vi "Get QControl Class Hierarchy.vi"(11 "ControlClassWizard in":refnum<class "QControl Creation Wizard.lvclass">) -> (0 "error out":errorcluster, 2 "QControl Class Hierarchy":string[][](array[string]), 3 "ControlClassWizard out":refnum<class "QControl Creation Wizard.lvclass">)   [LabVIEW 2015, in "QControl Creation Wizard.lvclass"]
doc: "<b> </b> <b> </b>\n©2016 Q Software Innovations, LLC (QSI)\nwritten by Quentin Alldredge\nproduced in LabVIEW 2015\n\nsupport@qsoftwareinnovations.com\nwww.qsoftwareinnovations.com\n\nAll rights reserved.\n\nRedistribution and use in source and binary forms, with or without modification, are permitted provided that the following conditions are met:\n\n * Redistributions of source code must retain the above copyright notice, this list of conditions and the following disclaimer.\n * Redistributions in binary form must reproduce the above copyright notice, this list of conditions and the following disclaimer in the documentation and/or other materials provided with the distribution.\n * Neither the name of Q Software Innovations, LLC. nor the names of its contributors may be used to endorse or promote products derived from this software without specific prior written permission.\n\nTHIS SOFTWARE IS PROVIDED BY THE COPYRIGHT HOLDERS AND CONTRIBUTORS \"AS IS\" AND ANY EXPRESS OR IMPLIED WARRANTIES, INCLUDING, BUT NOT LIMITED TO, THE IMPLIED WARRANTIES OF MERCHANTABILITY AND FITNESS FOR A PARTICULAR PURPOSE ARE DISCLAIMED. IN NO EVENT SHALL THE COPYRIGHT OWNER OR CONTRIBUTORS BE LIABLE FOR ANY DIRECT, INDIRECT, INCIDENTAL, SPECIAL, EXEMPLARY, OR CONSEQUENTIAL DAMAGES (INCLUDING, BUT NOT LIMITED TO, PROCUREMENT OF SUBSTITUTE GOODS OR SERVICES; LOSS OF USE, DATA, OR PROFITS; OR BUSINESS INTERRUPTION) HOWEVER CAUSED AND ON ANY THEORY OF LIABILITY, WHETHER IN CONTRACT, STRICT LIABILITY, OR TORT (INCLUDING NEGLIGENCE OR OTHERWISE) ARISING IN ANY WAY OUT OF THE USE OF THIS SOFTWARE, EVEN IF ADVISED OF THE POSSIBILITY OF SUCH DAMAGE."
uses:
  QControl Creation Wizard.lvclass
  QControl Classes/Control/Control.lvclass
  QControl Creation Wizard.lvclass/QControl Creation Wizard.ctl
  New QControl Info/New QControl Info.lvclass/New QControl Info.ctl
  New QControl Info/Read App Refnum.vi
  New QControl Info/New QControl Info.lvclass
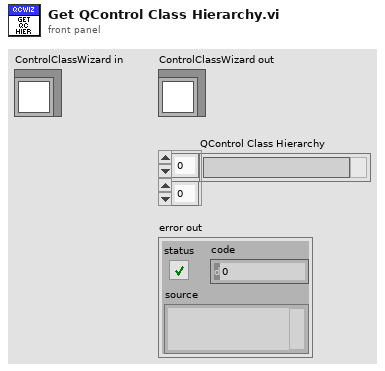
[diagram p1: front panel]
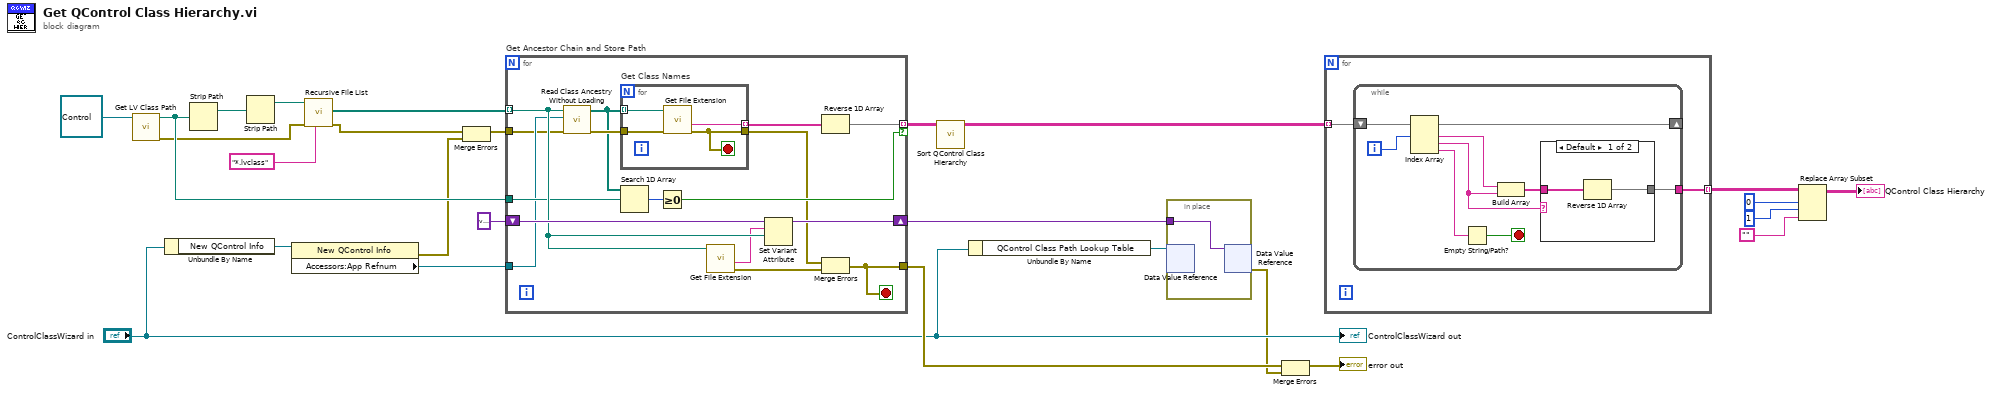
[diagram p0: block diagram]
diagram:
  n1 = call <vilib>:"Get LV Class Path.vi"("object"=refnum<class "Control.lvclass"> refnum ("Control")) -> ("error out"=w10:errorcluster, "class path"=w13:path)  [unwired: 9 in]
  n2 = Unbundle By Name("ControlClassWizard in") -> ("New QControl Info"=w14:refnum<data-value>)
  n3 = Strip Path(path=w13) -> (stripped path=w12:path)  [unwired: 1 out]
  n4 = Strip Path(path=w12) -> (stripped path=w15:path)  [unwired: 1 out]
  n5 = property class="New QControl Info"(reference=w14) -> (error out=w7:errorcluster, "Accessors:App Refnum"=w11:refnum<vi>)  [unwired: 1 in, 1 out]
  n6 = call <vilib>:"Recursive File List.vi"("pattern"="*.lvclass", "error in (no error)"=w10, "Folder Path"=w15) -> ("error out"=w9:errorcluster, "All Files in Dir"=w25:path[])  [unwired: 4 in, 3 out]
  n7 = Merge Errors(w9, w7) -> (w8:errorcluster)
  n8 = for "Get Ancestor Chain and Store Path" {
    tunnel: w25 -> [w37] mode=indexing
    tunnel: [w40] -> w24 mode=indexing if=w32
    shift-right: [w38] -> w2
    shift-left: variant -> [w39]
    tunnel: w13 -> [w34]
    tunnel: w11 -> [w31]
    tunnel: w8 -> [w30]
    tunnel: [w27] -> w6
    stop <- w27 stop-if-true
    n9 = call <vilib>:"Read Class Ancestry Without Loading.vi"("error in (no error)"=w30, "App Reference (this app)"=w31, "LabVIEW Class Path"=w37) -> ("error out"=w42:errorcluster, "Class Ancestry"=w35:path[])  [unwired: 7 in]
    n10 = for "Get Class Names" {
      tunnel: w42 -> [w46]
      tunnel: w35 -> [w45] mode=indexing
      tunnel: [w44] -> w41 mode=indexing
      tunnel: [w43] -> w28
      stop <- w43 stop-if-true
      n11 = call <vilib>:"Get File Extension.vi"("error in (no error)"=w46, "file"=w45) -> ("error out"=w43:errorcluster, "filename without extension"=w44:string)  [unwired: 5 in, 3 out]
    }
    n12 = Search 1D Array(1D array=w35, element=w34) -> (index of element=w33:i32)  [unwired: 1 in]
    n13 = Greater Or Equal To 0?(x=w33) -> (x >= 0?=w32:bool)
    n14 = call <vilib>:"Get File Extension.vi"("file"=w37) -> ("error out"=w29:errorcluster, "filename without extension"=w36:string)  [unwired: 6 in, 3 out]
    n15 = Set Variant Attribute(Variant=w39, name=w36, value=w37) -> (Variant out=w38:variant)  [unwired: 1 in, 2 out]
    n16 = Reverse 1D Array(array=w41) -> (reversed array=w40:string[])
    n17 = Merge Errors(w28, w29) -> (w27:errorcluster)
  }
  n18 = call "Sort QControl Class Hierarchy.vi"("Class List in"=w24) -> ("Class List out"=w23:string[][])  [unwired: 10 in]
  n19 = Unbundle By Name("ControlClassWizard in") -> ("QControl Class Path Lookup Table"=w3:refnum<data-value>)
  n20 = in-place {
    in-place-border: w2 -> [w47]
    n21 = in-place-dvr #1(w3) -> ()  [unwired: 2 out]
    n22 = in-place-dvr #1(w47) -> (w1:errorcluster)  [unwired: 1 out]
  }
  n23 = Merge Errors(w6, w1) -> (→"error out":errorcluster)
  n24 = for {
    tunnel: w23 -> [w49] mode=indexing
    tunnel: [w48] -> w22 mode=indexing
    n25 = while {
      shift-right: [w57] -> _
      shift-left: w49 -> [w57]
      tunnel: [w50] -> w48
      i -> [w56]
      stop <- w54 stop-if-true
      n26 = Index Array(array=w57, index #1=w56) -> (element #1=w51:string, element #2=w53:string, element #3=w55:string)  [unwired: 2 in]
      n27 = Empty String/Path?(string/path=w55) -> (empty?=w54:bool)
      n28 = Build Array(w51, w53) -> (w52:string[])
      n29 = case shown="Default" w53 {
        tunnel: w52 -> [w59 w60]
        tunnel: [w58 w60] -> w50
        frame Default {
          n30 = Reverse 1D Array(array=w59) -> (reversed array=w58:string[])
        }
        frame "" {
        }
      }
    }
  }
  n31 = Replace Array Subset(array=w22, new element="", index (row)=0, index (col)=1 ("disabled index (col)")) -> (→"QControl Class Hierarchy":string[][])
  "ControlClassWizard out" <- "ControlClassWizard in"
